vi "GUI_StagingMagSpec.vi"() -> ()   [LabVIEW 2013]
uses:
  Device Driver/shared/OnOffTypeDef.ctl
  shared programs/GUI_Template/GUI_master/tcp new data cluster.ctl
  <vilib>/Waveform/WDTOps.llb/WDT Waveform to XY Pairs DBL.vi
  <vilib>/vision/NI_Vision_Development_Module.lvlib
panel:
  in  "save ref":bool
  in  "log E lineout":bool
  out "XY Graph 2":cluster{dbl[], dbl[]}[](graph)
  out "XY Graph":cluster{dbl[], dbl[]}(graph)
  out "dgh":waveform(dbl)(graph) caption="Spectrum"
  out "charge":dbl(graph)
  in  "camsettings.cam 2.center::1":dbl=68.0 caption="center" min=0.0 max=500.0
  in  "camsettings.cam 0.center::1":dbl=68.0 caption="center" min=0.0 max=600.0
  out "MagCam3::1":T1(plugin-control) caption="MagCam3"
  out "MagCam1::1":T1(plugin-control) caption="MagCam1"
  out "MagCam2::1":T1(plugin-control) caption="MagCam2"
  in  "Trigger::1":T2 caption="Trigger"
  in  "exposure::1":dbl=63.593734 caption="exposure" min=0.01 max=0.1 format="%#_6p"
  in  "camsettings.cam 1.center::1":dbl=68.0 caption="center" min=0.0 max=500.0
  in  "ROIstring::1":string="cam 1>>68>>14>>682>>116" caption="ROIString::1"
  out "image":T1(plugin-control)
  in  "profile::1":waveform(dbl)[](graph)=[{"t0"=timestamp(0 s since 1904-01-01), "dt"=0.1, "Y"=array[401 elements]}] caption="Spectrum"
  in  "Save::1":T2 caption="Save"
  out "Bfield::1":dbl caption="Bfiled [mT]" min=0.0 max=0.0
  out "maxEnergy::1":dbl caption="maxEnergy" min=0.0 max=0.0
  out "peakEnergy(max)::1":dbl=63.593734 caption="peak energy(max)" min=0.0 max=0.0
  out "peakEnergy(min)::1":dbl=25.593734 caption="peak energy(min)" min=0.0 max=0.0
  in  "spectrum::1":waveform(dbl)[](graph)=[{"t0"=timestamp(0 s since 1904-01-01), "dt"=0.1, "Y"=array[639 elements]}] caption="Spectrum"
  out "GUIdevice 2":string="StagingHallProbe"
  out "image::1":T1(plugin-control) caption="image"
  out "mean::1":dbl=42.826821 caption="mean" min=0.0 max=0.0
  in  "Select device":string(combo)="StagingMagSpec"
  in  "Refresh Button":bool
  in  "charge::1":dbl=28.630916 caption="charge" min=0.0 max=0.0
  out "device status::1":string="Initialized" caption="Status"
  in  "stop":bool=TRUE
  out "GUIdevice 1":string="StagingMagSpec"
  out "UDP error message":string
  # "Staging Magnetic Spectrometer"
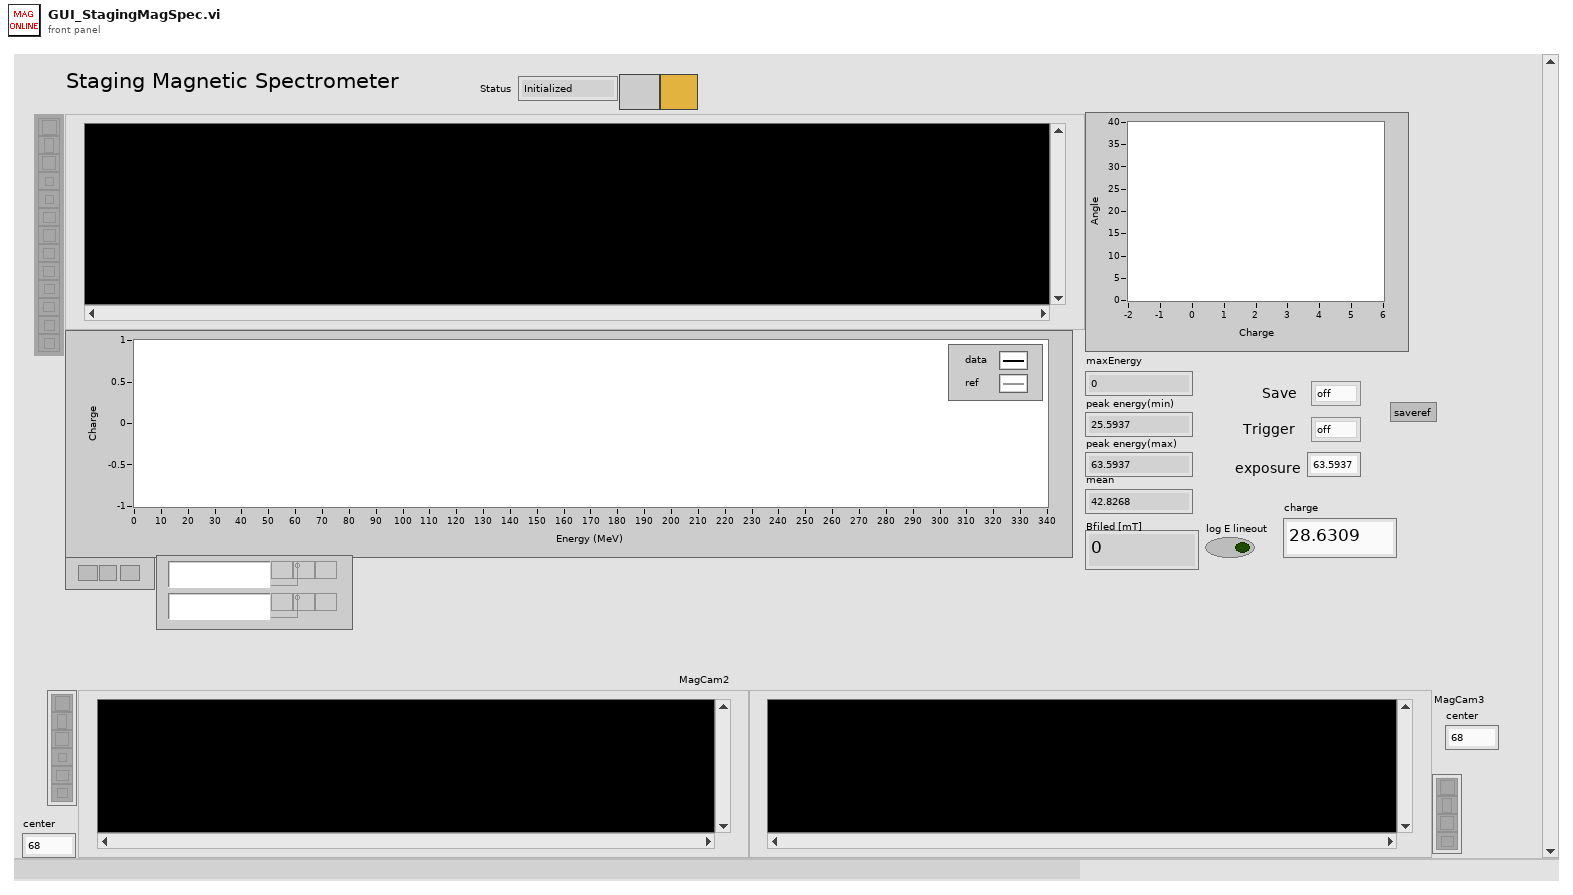
[diagram p1: front panel]
types:
  T1 = typedef "IMAQ Image.ctl" = refnum<image>
  T2 = typedef "OnOffTypeDef.ctl" = enum16{"off", "on"}
  T3 = typedef "Image Type" = u32
  T4 = typedef "tcp new data cluster.ctl" = cluster{"EventEnum":enum16{"new data", "connection status update"}, "Device name":string}
  T5 = cluster{"Starting Value":sgl, "Incremental Value":sgl, "Histogram":u32[]}
  T6 = cluster{"Global Rectangle":i32[], "Contours":cluster{"Contour Type":u32, "ROI Type":u32, "Points":i32[]}[]}
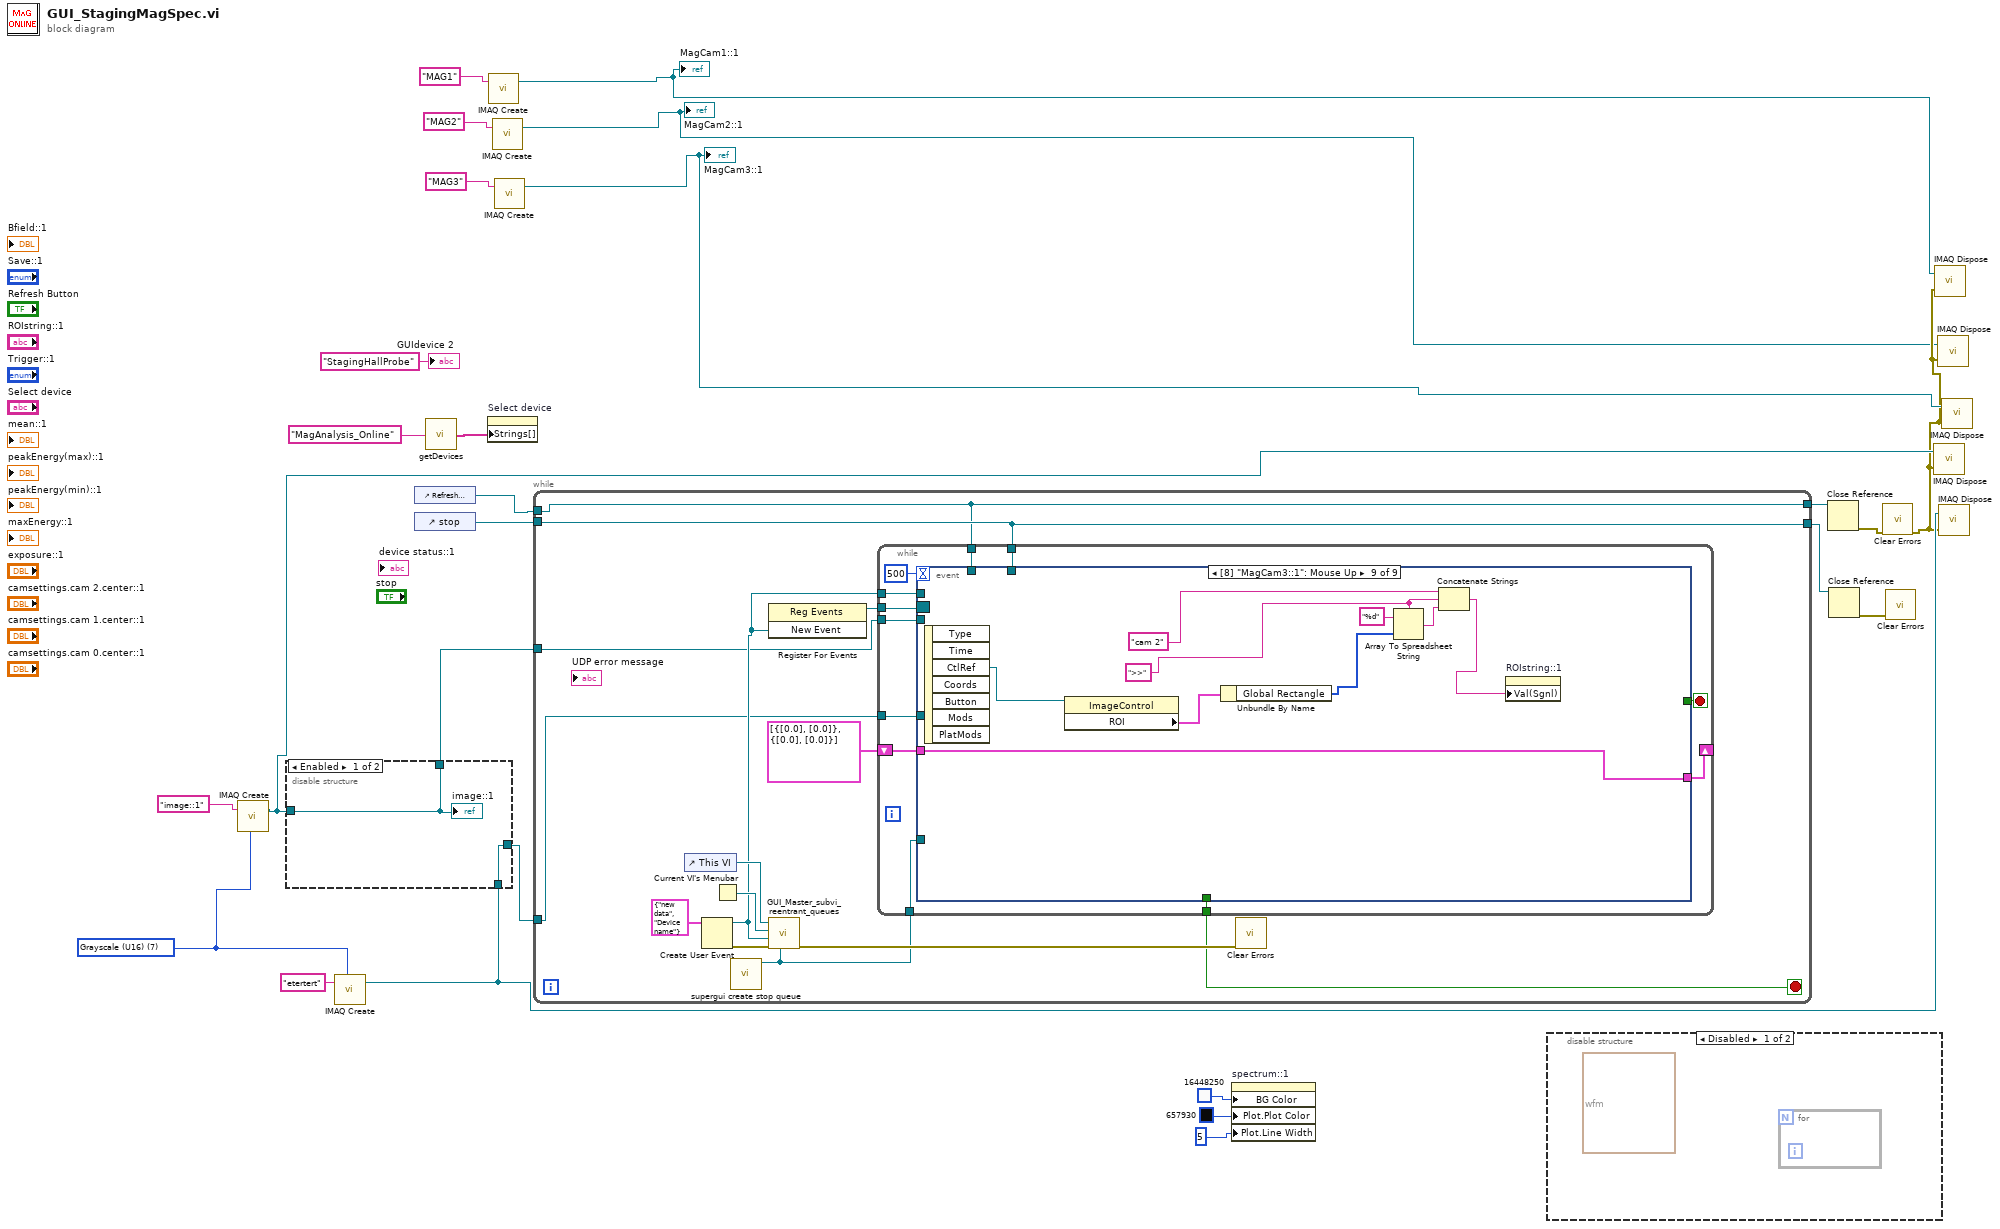
[diagram p0: block diagram]
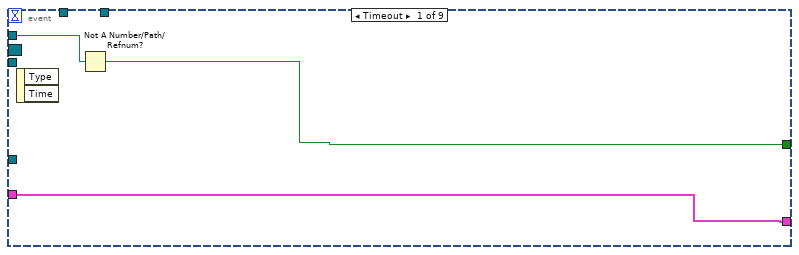
[diagram p4: hidden frame]
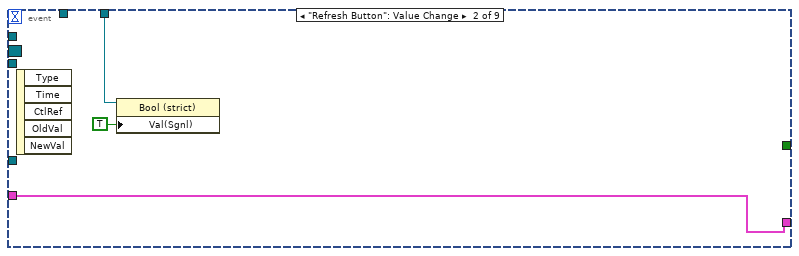
[diagram p5: hidden frame]
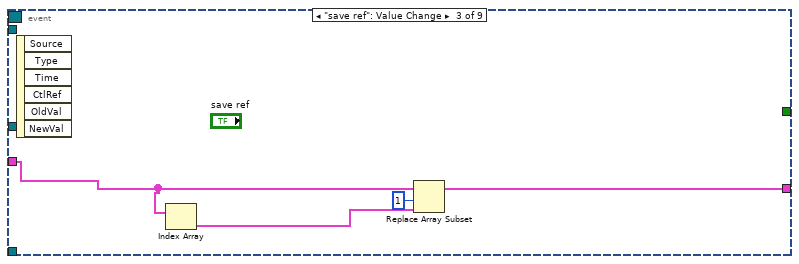
[diagram p6: hidden frame]
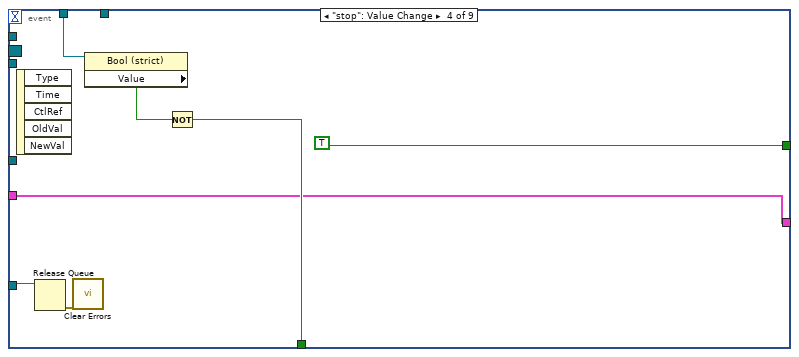
[diagram p7: hidden frame]
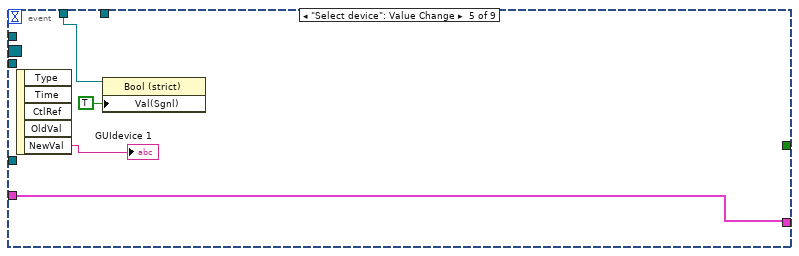
[diagram p8: hidden frame]
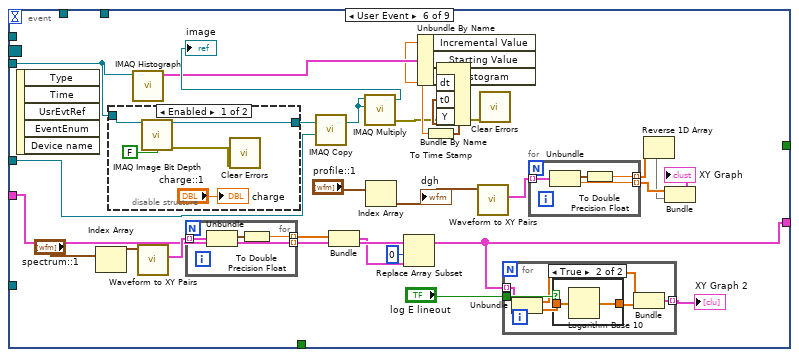
[diagram p9: hidden frame]
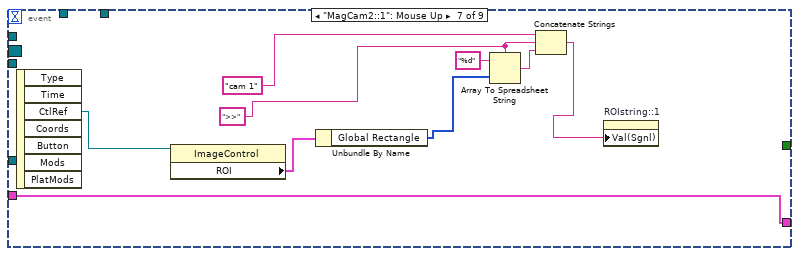
[diagram p12: hidden frame]
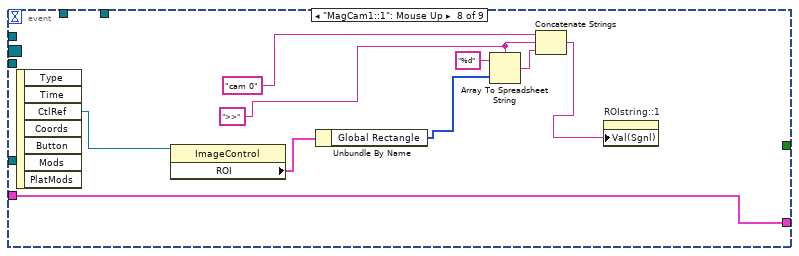
[diagram p13: hidden frame]
diagram:
  w11 = T3 7 items=["Grayscale (U8)", "Grayscale (I16)", "Grayscale (SGL)", "Complex (CSG)", "RGB (U32)", "HSL (U32)", "RGB (U64)", "Grayscale (U16)"] ("Image Type")
  n1 = call "IMAQ Create"("Image Name"="image::1", "Image Type"=w11) -> ("New Image"=w5:T1)  [unwired: 3 in, 1 out]
  n2 = call "IMAQ Create"("Image Name"="etertert", "Image Type"=w11) -> ("New Image"=w6:T1)  [unwired: 3 in, 1 out]
  n3 = disable-structure shown="Enabled" {
    disable-tunnel: [w27 _] -> w14
    disable-tunnel: [w28 _] -> w13
    disable-tunnel: w6 -> [w28 _]
    disable-tunnel: w5 -> [w27 _]
    frame Enabled {
      "image::1" <- w27
    }
    frame Disabled {
    }
  }
  n4 = control-ref of="Refresh Button"() -> (w24:refnum<vi>)
  n5 = control-ref of="stop"() -> (w26:refnum<vi>)
  n6 = call "getDevices.vi"("Device Class"="MagAnalysis_Online") -> ("All Devices"=w19:string[])
  n7 = property on="Select device" class="CmbBox"("Strings[]"=w19) -> ()  [unwired: 2 in, 2 out]
  n8 = call "IMAQ Create"("Image Name"="MAG1") -> ("New Image"=w1:T1)  [unwired: 4 in, 1 out]
  "MagCam1::1" <- w1
  n9 = call "IMAQ Create"("Image Name"="MAG2") -> ("New Image"=w2:T1)  [unwired: 4 in, 1 out]
  "MagCam2::1" <- w2
  n10 = call "IMAQ Create"("Image Name"="MAG3") -> ("New Image"=w4:T1)  [unwired: 4 in, 1 out]
  "MagCam3::1" <- w4
  n11 = while {
    tunnel: w26 -> [w35]
    tunnel: [w35] -> w25
    tunnel: w24 -> [w34]
    tunnel: [w34] -> w23
    tunnel: w14 -> [w32]
    tunnel: w13 -> [w31]
    stop <- w33 stop-if-true
    n12 = control-ref of="This VI"() -> (w42:refnum<vi>)
    n13 = Create User Event(user event datatype=T4 {"EventEnum"=enum."new data", "Device name"="Device name"} ("New Event")) -> (user event=w36:refnum<user-event>, error out=w39:errorcluster)  [unwired: 1 in]
    n14 = Current VI's Menubar() -> (w41:refnum<k9>)
    n15 = call "supergui create stop queue.vi"() -> ("STOP Queue out"=w29:refnum<queue>)  [unwired: 11 in]
    n16 = register-events(w36) -> (reference out=w37:refnum<event-registration>)  [unwired: 2 in, 1 out]
    n17 = call "GUI_Master_subvi_reentrant_queues.vi"("STOP Queue in"=w29, "error in (no error)"=w39, "tcp data event"=w36, "Caller menu reference"=w41, "Caller VI ref"=w42) -> ("error out"=w38:errorcluster)  [unwired: 6 in]
    n18 = while {
      tunnel: w37 -> [w54]
      tunnel: w36 -> [w51]
      tunnel: w35 -> [w50]
      tunnel: w34 -> [w49]
      tunnel: [w46] -> w33
      tunnel: w32 -> [w48]
      tunnel: w31 -> [w47]
      shift-right: [w44] -> _
      shift-left: cluster{dbl[], dbl[]}[] [{[0.0], [0.0]}, {[0.0], [0.0]}] ("ref") -> [w45]
      tunnel: w29 -> [w43]
      stop <- w53 stop-if-true
      n19 = event shown="[8] \"MagCam3::1\": Mouse Up" {
        selector: w54 -> [_ _ _ _ _ _ _ _ _]
        dyn-events: _ -> [_ _ _ _ _ _ _ _ _]
        timeout: 500 -> [_ _ _ _ _ _ _ _ _]
        tunnel: [w56 _ _ TRUE _ _ _ _ _] -> w53
        tunnel: w51 -> [w57 _ _ _ _ _ _ _ _]
        tunnel: w50 -> [_ w59 _ _ _ _ _ _ _]
        tunnel: w49 -> [_ _ _ w71 w74 _ _ _ _]
        tunnel: [_ _ _ w69 _ _ _ _ _] -> w46
        tunnel: w48 -> [_ _ _ _ _ w96 _ _ _]
        tunnel: w47 -> [_ _ _ _ _ w104 _ _ _]
        tunnel: w45 -> [w55 w58 w62 w67 w72 w82 w128 w137 w146]
        tunnel: [w55 w58 w63 w67 w72 w77 w128 w137 w146] -> w44
        tunnel: w43 -> [_ _ _ w66 _ _ _ _ _]
        event Timeout {
          n20 = event-data() -> ()  [unwired: 1 in, 2 out]
          n21 = Not A Number/Path/Refnum?(number/path/refnum=w57) -> (NaN/Path/Refnum?=w56:bool)
        }
        event "Refresh Button": Value Change {
          n22 = event-data() -> ()  [unwired: 1 in, 5 out]
          n23 = property class="Bool (strict)"(reference=w59, "Val(Sgnl)"=TRUE ("Value (Signaling)")) -> ()  [unwired: 1 in, 2 out]
        }
        event "save ref": Value Change {
          n24 = event-data() -> ()  [unwired: 1 in, 6 out]
          n25 = Index Array(array=w62) -> (element=w61:cluster{dbl[], dbl[]})  [unwired: 1 in]
          n26 = Replace Array Subset(array=w62, new element=w61, index=1) -> (w63:cluster{dbl[], dbl[]}[])
        }
        event "stop": Value Change {
          n27 = event-data() -> ()  [unwired: 1 in, 5 out]
          n28 = Release Queue(queue=w66) -> (error out=w65:errorcluster)  [unwired: 2 in, 2 out]
          n29 = call <vilib>:"Clear Errors.vi"("error in (no error)"=w65) -> ()  [unwired: 6 in, 1 out]
          n30 = property class="Bool (strict)"(reference=w71) -> ("Value"=w70:bool)  [unwired: 1 in, 2 out]
          n31 = Not(x=w70) -> (.not. x?=w69:bool)
        }
        event "Select device": Value Change {
          n32 = event-data() -> ("NewVal"=→"GUIdevice 1":string)  [unwired: 1 in, 4 out]
          n33 = property on="Property Node" class="Bool (strict)"(reference=w74, "Val(Sgnl)"=TRUE ("Value (Signaling)")) -> ()  [unwired: 1 in, 2 out]
        }
        event User Event {
          n34 = event-data() -> ()  [unwired: 1 in, 5 out]
          n35 = Index Array(array="spectrum::1") -> (element=w86:waveform(dbl))  [unwired: 1 in]
          n36 = disable-structure shown="Enabled" {
            disable-tunnel: w96 -> [w126 w127]
            disable-tunnel: [w125 w127] -> w95
            frame Enabled {
              n37 = call "IMAQ Image Bit Depth"("Image"=w126, "Get/Set Bit Depth? (Set)"=FALSE) -> ("Image Out"=w125:T1, "error out"=w122:errorcluster)  [unwired: 11 in, 1 out]
              n38 = call <vilib>:"Clear Errors.vi"("error in (no error)"=w122) -> ()  [unwired: 6 in, 1 out]
              "charge" <- "charge::1"
            }
            frame Disabled {
            }
          }
          n39 = call "IMAQ Histograph"("Image"=w96) -> ("Histogram Graph"=w101:T5)  [unwired: 7 in, 3 out]
          n40 = call-poly <vilib>:"Waveform to XY Pairs.vi"("waveform in"=w86) -> ("XY pairs"=w85:cluster{"x":timestamp, "y":dbl}[])  [unwired: 8 in, 2 out]
          n41 = for {
            tunnel: w85 -> [w117] mode=indexing
            tunnel: [w115] -> w83 mode=indexing
            tunnel: [w114] -> w79 mode=indexing
            n42 = Unbundle(w117) -> ("x"=w116:timestamp, "y"=w114:dbl)
            n43 = To Double Precision Float(number=w116) -> (double precision float=w115:dbl)
          }
          n44 = call "IMAQ Copy"("Image Dst"=w104, "Image Src"=w95) -> ("Image Dst Out"=w103:T1)  [unwired: 4 in, 1 out]
          n45 = Bundle(w83, w79) -> (w80:cluster{dbl[], dbl[]})  [unwired: 1 in]
          n46 = call "IMAQ Multiply"("Image Src A"=w103, "Image Dst"=w103) -> ("Image Dst Out"=→"image":T1, "error out"=w94:errorcluster)  [unwired: 5 in]
          n47 = Index Array(array="profile::1") -> (element=w92:waveform(dbl))  [unwired: 1 in]
          "dgh" <- w92
          n48 = Replace Array Subset(array=w82, new element=w80, index=0) -> (w77:cluster{dbl[], dbl[]}[])
          n49 = Unbundle By Name(w101) -> ("Incremental Value"=w100:sgl, "Starting Value"=w99:sgl, "Histogram"=w97:u32[])
          n50 = To Time Stamp(1:w99) -> (0:w98:timestamp)
          n51 = Bundle By Name("dt"=w100, "t0"=w98, "Y"=w97) -> ()  [unwired: 1 in, 1 out]
          n52 = call-poly <vilib>:"Waveform to XY Pairs.vi"("waveform in"=w92) -> ("XY pairs"=w91:cluster{"x":timestamp, "y":dbl}[])  [unwired: 8 in, 2 out]
          n53 = call <vilib>:"Clear Errors.vi"("error in (no error)"=w94) -> ()  [unwired: 6 in, 1 out]
          n54 = for {
            tunnel: "log E lineout" -> [w110]
            tunnel: w77 -> [w108] mode=indexing
            tunnel: [w105] -> w76 mode=indexing
            n55 = Unbundle(w108) -> (w106:dbl[], w109:dbl[])
            n56 = case shown="True" w110 {
              tunnel: w109 -> [w111 w113]
              tunnel: [w111 w112] -> w107
              frame False {
              }
              frame True {
                n57 = Logarithm Base 10(1:w113) -> (0:w112:dbl[])
              }
            }
            n58 = Bundle(w106, w107) -> (w105:cluster{dbl[], dbl[]})  [unwired: 1 in]
          }
          "XY Graph 2" <- w76
          n59 = for {
            tunnel: w91 -> [w121] mode=indexing
            tunnel: [w119] -> w88 mode=indexing
            tunnel: [w118] -> w89 mode=indexing
            n60 = Unbundle(w121) -> ("x"=w120:timestamp, "y"=w118:dbl)
            n61 = To Double Precision Float(number=w120) -> (double precision float=w119:dbl)
          }
          n62 = Reverse 1D Array(array=w88) -> (reversed array=w87:dbl[])
          n63 = Bundle(w89, w87) -> (→"XY Graph":cluster{dbl[], dbl[]})  [unwired: 1 in]
        }
        event "MagCam2::1": Mouse Up {
          w132 = ">>"
          n64 = event-data() -> ("CtlRef"=w129:refnum<vi>)  [unwired: 1 in, 6 out]
          n65 = property class="ImageControl"(reference=w129) -> ("ROI"=w136:T6)  [unwired: 1 in, 2 out]
          n66 = Unbundle By Name(w136) -> ("Global Rectangle"=w135:i32[])
          n67 = Array To Spreadsheet String(delimiter (Tab)=w132, array=w135, 3:"%d" ("format string")) -> (spreadsheet string=w131:string)
          n68 = Concatenate Strings("cam 1", w132, w131) -> (w130:string)
          n69 = property on="ROIstring::1" class="Str"("Val(Sgnl)"=w130) -> ()  [unwired: 2 in, 2 out]
        }
        event "MagCam1::1": Mouse Up {
          w141 = ">>"
          n70 = event-data() -> ("CtlRef"=w138:refnum<vi>)  [unwired: 1 in, 6 out]
          n71 = property class="ImageControl"(reference=w138) -> ("ROI"=w145:T6)  [unwired: 1 in, 2 out]
          n72 = Unbundle By Name(w145) -> ("Global Rectangle"=w144:i32[])
          n73 = Array To Spreadsheet String(delimiter (Tab)=w141, array=w144, 3:"%d" ("format string")) -> (spreadsheet string=w140:string)
          n74 = Concatenate Strings("cam 0", w141, w140) -> (w139:string)
          n75 = property on="ROIstring::1" class="Str"("Val(Sgnl)"=w139) -> ()  [unwired: 2 in, 2 out]
        }
        event "MagCam3::1": Mouse Up {
          w150 = ">>"
          n76 = event-data() -> ("CtlRef"=w147:refnum<vi>)  [unwired: 1 in, 6 out]
          n77 = property class="ImageControl"(reference=w147) -> ("ROI"=w154:T6)  [unwired: 1 in, 2 out]
          n78 = Unbundle By Name(w154) -> ("Global Rectangle"=w153:i32[])
          n79 = Array To Spreadsheet String(delimiter (Tab)=w150, array=w153, 3:"%d" ("format string")) -> (spreadsheet string=w149:string)
          n80 = Concatenate Strings("cam 2", w150, w149) -> (w148:string)
          n81 = property on="ROIstring::1" class="Str"("Val(Sgnl)"=w148) -> ()  [unwired: 2 in, 2 out]
        }
      }
    }
    n82 = call <vilib>:"Clear Errors.vi"("error in (no error)"=w38) -> ()  [unwired: 6 in, 1 out]
  }
  n83 = property on="spectrum::1" class="WFGraph (strict)"("BG Color"=u32 16448250, "Plot.Plot Color"=u32 657930, "Plot.Line Width"=u8 5) -> ()  [unwired: 2 in, 2 out]
  n84 = disable-structure shown="Disabled" {
    frame Disabled {
      (unwired) waveform(dbl) {"t0"=timestamp(0 s since 1904-01-01), "dt"=1.0, "Y"=[]} ("Waveform")
      n85 = for {
      }
    }
    frame Enabled {
    }
  }
  n86 = Close Reference(reference=w23) -> (error out=w22:errorcluster)  [unwired: 1 in]
  n87 = Close Reference(reference=w25) -> (error out=w21:errorcluster)  [unwired: 1 in]
  n88 = call <vilib>:"Clear Errors.vi"("error in (no error)"=w22) -> ("error out"=w3:errorcluster)  [unwired: 6 in]
  n89 = call <vilib>:"Clear Errors.vi"("error in (no error)"=w21) -> ()  [unwired: 6 in, 1 out]
  n90 = call "IMAQ Dispose"("Image"=w5, "error in (no error)"=w3) -> ()  [unwired: 4 in, 1 out]
  n91 = call "IMAQ Dispose"("Image"=w1, "error in (no error)"=w3) -> ()  [unwired: 4 in, 1 out]
  n92 = call "IMAQ Dispose"("Image"=w2, "error in (no error)"=w3) -> ()  [unwired: 4 in, 1 out]
  n93 = call "IMAQ Dispose"("Image"=w6, "error in (no error)"=w3) -> ()  [unwired: 4 in, 1 out]
  n94 = call "IMAQ Dispose"("Image"=w4, "error in (no error)"=w3) -> ()  [unwired: 4 in, 1 out]
  "GUIdevice 2" <- "StagingHallProbe" ("GUIdevice 2")
